vi "7495_Fast2.vi"(4 "Clk 1\nR-Shift":bool, 5 "Serial\nInput":bool, 6 "Clk 2\nL-Shift":bool, 7 "Mode\nControl":bool, 8 "D":bool, 9 "C":bool, 10 "B":bool, 11 "A":bool) -> (0 "OD":bool, 1 "OC":bool, 2 "OB":bool, 3 "OA":bool)   [LabVIEW 2012]
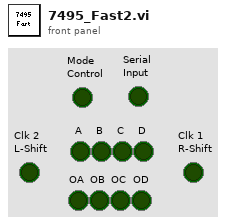
[diagram p1: front panel]
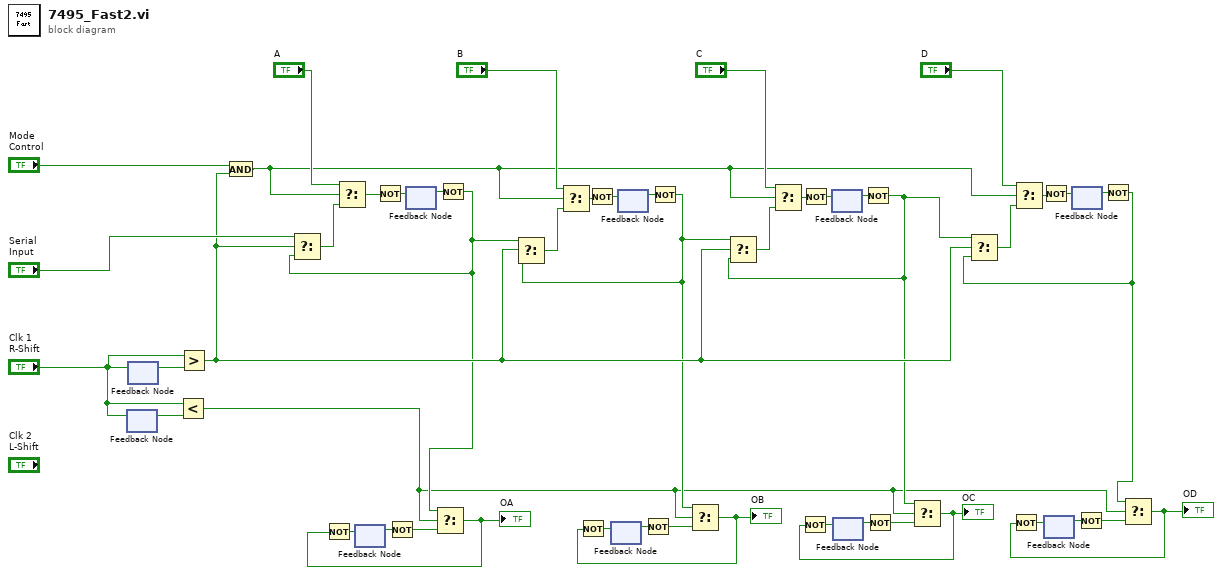
[diagram p0: block diagram]
diagram:
  n1 = feedback #1() -> (w18:bool)  [unwired: 1 in]
  n2 = feedback-in #1("Clk 1\nR-Shift") -> ()
  n3 = feedback #2() -> (w38:bool)  [unwired: 1 in]
  n4 = feedback-in #2("Clk 1\nR-Shift") -> ()
  n5 = Less?(x="Clk 1\nR-Shift", y=w18) -> (x < y?=w1:bool)
  n6 = Greater?(x="Clk 1\nR-Shift", y=w38) -> (0:w29:bool)
  n7 = And(x="Mode\nControl", y=w29) -> (x .and. y?=w28:bool)
  n8 = feedback #3() -> (w23:bool)  [unwired: 1 in]
  n9 = Not(x=w23) -> (.not. x?=w21:bool)
  n10 = feedback #4() -> (w36:bool)  [unwired: 1 in]
  n11 = Not(x=w36) -> (.not. x?=w19:bool)
  n12 = Select(t="Serial\nInput", s=w29, f=w19) -> (s? t:f=w39:bool)
  n13 = Select(t="A", s=w28, f=w39) -> (s? t:f=w27:bool)
  n14 = Not(x=w27) -> (.not. x?=w37:bool)
  n15 = feedback-in #4(w37) -> ()
  n16 = Select(t=w19, s=w1, f=w21) -> (s? t:f=w20:bool)
  "OA" <- w20
  n17 = Not(x=w20) -> (.not. x?=w22:bool)
  n18 = feedback-in #3(w22) -> ()
  n19 = feedback #5() -> (w14:bool)  [unwired: 1 in]
  n20 = feedback #6() -> (w35:bool)  [unwired: 1 in]
  n21 = Not(x=w14) -> (.not. x?=w16:bool)
  n22 = Not(x=w35) -> (.not. x?=w12:bool)
  n23 = Select(t=w19, s=w29, f=w12) -> (s? t:f=w42:bool)
  n24 = Select(t="B", s=w28, f=w42) -> (s? t:f=w26:bool)
  n25 = Not(x=w26) -> (.not. x?=w34:bool)
  n26 = feedback-in #6(w34) -> ()
  n27 = Select(t=w12, s=w1, f=w16) -> (s? t:f=w13:bool)
  "OB" <- w13
  n28 = Not(x=w13) -> (.not. x?=w15:bool)
  n29 = feedback-in #5(w15) -> ()
  n30 = feedback #7() -> (w32:bool)  [unwired: 1 in]
  n31 = feedback #8() -> (w11:bool)  [unwired: 1 in]
  n32 = Not(x=w32) -> (.not. x?=w8:bool)
  n33 = Select(t=w12, s=w29, f=w8) -> (s? t:f=w41:bool)
  n34 = Select(t="C", s=w28, f=w41) -> (s? t:f=w25:bool)
  n35 = Not(x=w25) -> (.not. x?=w33:bool)
  n36 = feedback-in #7(w33) -> ()
  n37 = Not(x=w11) -> (.not. x?=w9:bool)
  n38 = Select(t=w8, s=w1, f=w9) -> (s? t:f=w7:bool)
  "OC" <- w7
  n39 = Not(x=w7) -> (.not. x?=w10:bool)
  n40 = feedback-in #8(w10) -> ()
  n41 = feedback #9() -> (w4:bool)  [unwired: 1 in]
  n42 = feedback #10() -> (w31:bool)  [unwired: 1 in]
  n43 = Not(x=w4) -> (.not. x?=w6:bool)
  n44 = Not(x=w31) -> (.not. x?=w2:bool)
  n45 = Select(t=w8, s=w29, f=w2) -> (s? t:f=w40:bool)
  n46 = Select(t="D", s=w28, f=w40) -> (s? t:f=w24:bool)
  n47 = Not(x=w24) -> (.not. x?=w30:bool)
  n48 = feedback-in #10(w30) -> ()
  n49 = Select(t=w2, s=w1, f=w6) -> (s? t:f=w3:bool)
  "OD" <- w3
  n50 = Not(x=w3) -> (.not. x?=w5:bool)
  n51 = feedback-in #9(w5) -> ()
